vi "DeviceDemo.vi"() -> ()   [LabVIEW 2020]
uses:
  lib/SnapMB.lvlib
panel:
  out "Error":string="No Error"
  out "Holding Regs":u16[](array[numeric])
  out "error out":errorcluster
  in  "stop":bool
  out "Log":string
  in  "Device ID":u8=1
  in  "Port":u16=502
  in  "Proto":i32(ring) items=["TCP", "UDP", "RTUOverTCP", "RTUOverUDP"]
  in  "Address":string="127.0.0.1"
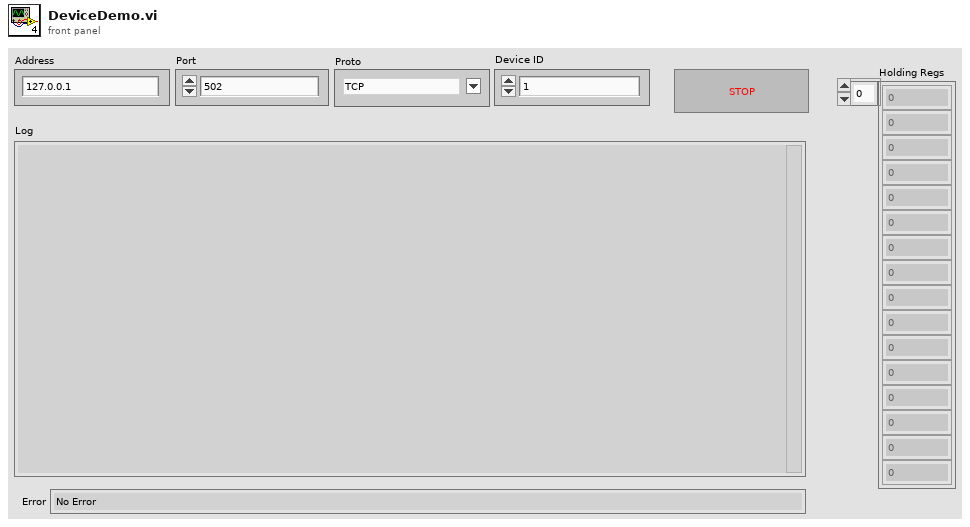
[diagram p1: front panel]
types:
  T1 = enum16{"Discrete Inputs", "Coils", "Input Registers", "Holding Registers"}
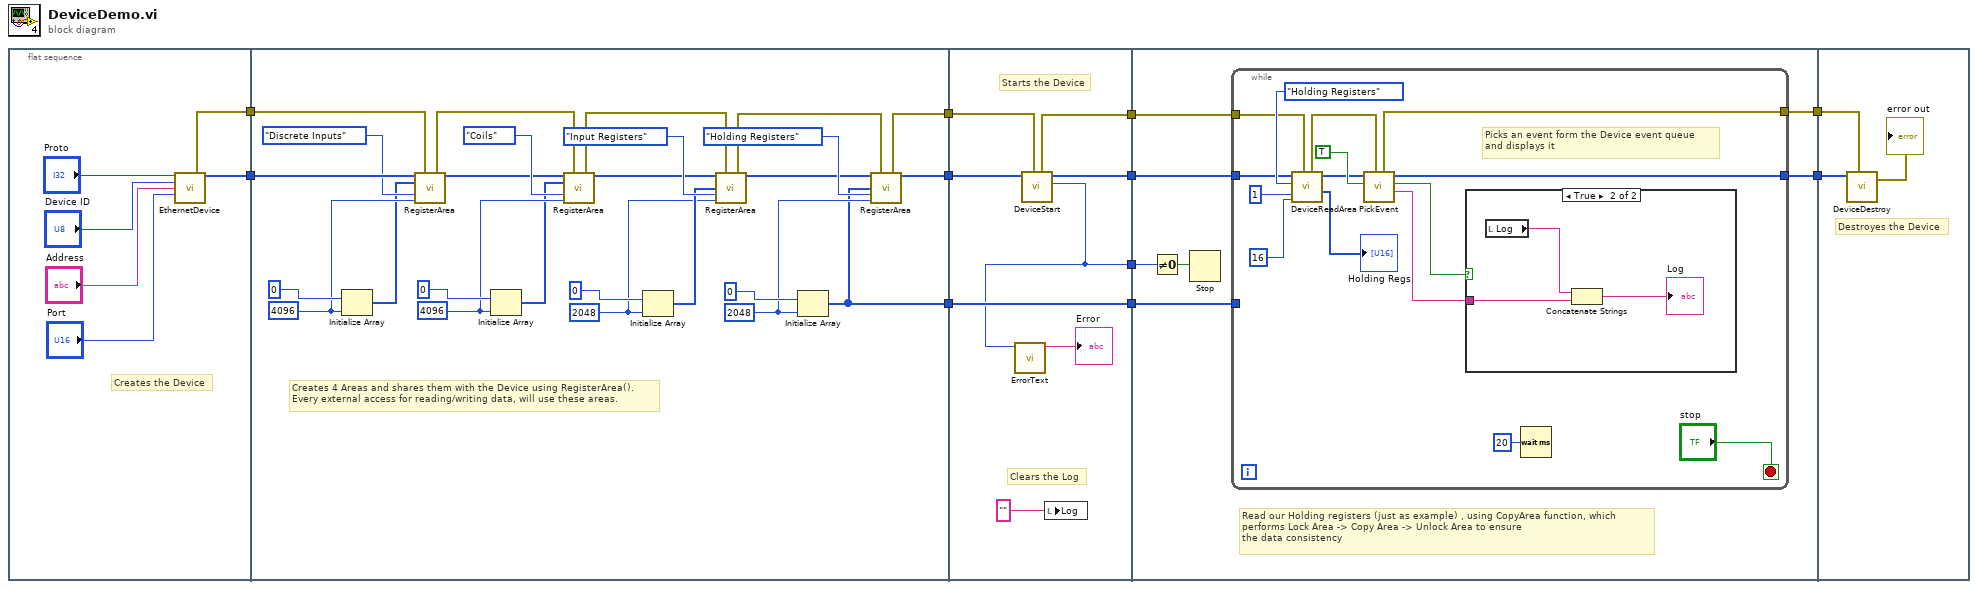
[diagram p0: block diagram]
diagram:
  n1 = flat-sequence {
    tunnel: [w13] -> w11
    tunnel: [w12] -> w9
    tunnel: w11 -> [w42]
    tunnel: [w24] -> w10
    tunnel: w9 -> [w23]
    tunnel: [w19] -> w8
    tunnel: [w18] -> w1
    tunnel: w10 -> [w51]
    tunnel: w8 -> [w50]
    tunnel: [w49] -> w7
    tunnel: [w44] -> w6
    tunnel: [w48] -> w5
    tunnel: [w47] -> w2
    tunnel: w1 -> [w47]
    tunnel: w7 -> [w58]
    tunnel: w6 -> [w56]
    tunnel: w5 -> [w55]
    tunnel: [w54] -> w4
    tunnel: [w53] -> w3
    tunnel: w2 -> [w52]
    tunnel: w4 -> [w79]
    tunnel: w3 -> [w78]
    frame #0 {
      # "Creates the Device"
      n2 = call "EthernetDevice.vi"("Proto"="Proto", "DeviceID"="Device ID", "Address"="Address", "Port"="Port") -> ("error out"=w12:errorcluster, "Device"=w13:u64[])  [unwired: 10 in]
    }
    frame #1 {
      w25 = 2048 ("dimension size")
      w29 = 2048
      w37 = 4096
      w41 = 4096
      # "Creates 4 Areas and shares them with the Device using RegisterArea().\nEvery external access for reading/writing data, will use these areas."
      n3 = Initialize Array(u8 0, w41) -> (w39:u8[])
      n4 = call "RegisterArea.vi"("Handle In"=w42, "error in (no error)"=w23, "BitArea"=w39, "AreaID"=T1."Discrete Inputs", "Amount"=w41) -> ("error out"=w22:errorcluster, "Handle Out"=w34:u64[])  [unwired: 8 in, 1 out]
      n5 = Initialize Array(u8 0, w37) -> (w35:u8[])
      n6 = call "RegisterArea.vi"("Handle In"=w34, "error in (no error)"=w22, "BitArea"=w35, "AreaID"=T1."Coils", "Amount"=w37) -> ("error out"=w21:errorcluster, "Handle Out"=w30:u64[])  [unwired: 8 in, 1 out]
      n7 = Initialize Array(u16 0, w29) -> (w31:u16[])
      n8 = call "RegisterArea.vi"("Handle In"=w30, "error in (no error)"=w21, "WordArea"=w31, "AreaID"=T1."Input Registers", "Amount"=w29) -> ("error out"=w20:errorcluster, "Handle Out"=w27:u64[])  [unwired: 8 in, 1 out]
      n9 = Initialize Array(u16 0 ("element"), w25) -> (w18:u16[])
      n10 = call "RegisterArea.vi"("Handle In"=w27, "error in (no error)"=w20, "WordArea"=w18, "AreaID"=T1."Holding Registers", "Amount"=w25) -> ("error out"=w19:errorcluster, "Handle Out"=w24:u64[])  [unwired: 8 in, 1 out]
    }
    frame #2 {
      # "Starts the Device"
      # "Clears the Log"
      n11 = call "DeviceStart.vi"("error in"=w50, "Handle In"=w51) -> ("Result"=w44:i32, "Handle Out"=w49:u64[], "error out"=w48:errorcluster)  [unwired: 7 in]
      n12 = call "ErrorText.vi"("ErrNo"=w44) -> ("ErrMessage"=→"Error":string)  [unwired: 9 in, 1 out]
      n13 = local write "Log"("" ("Log")) -> ()
    }
    frame #3 {
      # "Read our Holding registers (just as example) , using CopyArea function, which\nperforms Lock Area -> Copy Area -> Unlock Area to ensure\nthe data consistency"
      n14 = Not Equal To 0?(x=w56) -> (x != 0?=w57:bool)
      n15 = Stop(stop? (T)=w57) -> ()
      n16 = while {
        tunnel: w58 -> [w61]
        tunnel: w55 -> [w60]
        tunnel: [w68] -> w54
        tunnel: [w67] -> w53
        tunnel: w52 -> [_]
        stop <- "stop" stop-if-true
        # "Picks an event form the Device event queue \nand displays it"
        n17 = call "DeviceReadArea.vi"("error in (no error)"=w60, "Amount"=16, "Address"=u16 1, "AreaID"=T1."Holding Registers", "Handle In"=w61) -> ("Data"=→"Holding Regs":u16[], "Handle Out"=w62:u64[], "error out"=w59:errorcluster)  [unwired: 3 in, 1 out]
        n18 = call "PickEvent.vi"("error in (no error)"=w59, "CRLF"=TRUE, "Handle In"=w62) -> ("Text"=w71:string, "Picked"=w72:bool, "Handle Out"=w68:u64[], "error out"=w67:errorcluster)  [unwired: 5 in]
        n19 = case shown="True" w72 {
          tunnel: w71 -> [_ w74]
          frame False {
            # "No event picked : nothing to do"
          }
          frame True {
            n20 = local read "Log"() -> (w75:string)
            n21 = Concatenate Strings(w75, w74) -> (→"Log":string)
          }
        }
        n22 = Wait (ms)(milliseconds to wait=u32 20) -> ()  [unwired: 1 out]
      }
    }
    frame #4 {
      # "Destroyes the Device"
      n23 = call "DeviceDestroy.vi"("error in (no error)"=w78, "Handle In"=w79) -> ("error out"=→"error out":errorcluster)  [unwired: 9 in]
    }
  }
